vi "dfd_SOS Gain Distribution.vi"(7 "power of 2 initial?":bool, 9 "coefficients b":dbl[](array[numeric]), 10 "initial":dbl, 11 "norms":dbl[](array[numeric])) -> (0 "global gain":dbl, 1 "scaled coefficients b":dbl[](array[numeric]), 3 "input shift":i16)   [LabVIEW 2017, in "NI_DigFilter_FXP.lvlib"]
uses:
  <vilib>/addons/Digital Filter Design/NI_DigFilter_FXP.lvlib
  <vilib>/addons/Digital Filter Design/NI_DigFilterLicensed.lvlib
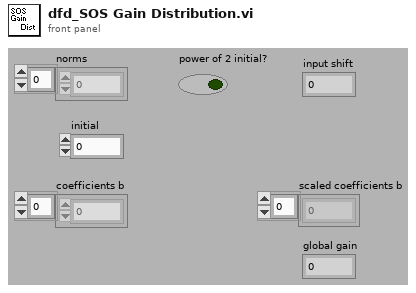
[diagram p1: front panel]
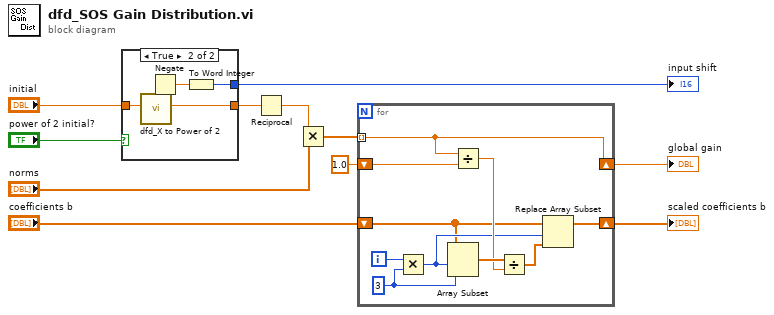
[diagram p0: block diagram]
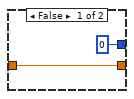
[diagram p2: hidden frame]
diagram:
  n1 = case shown="True" "power of 2 initial?" {
    tunnel: "initial" -> [w12 w18]
    tunnel: [i16 0 w15] -> w6
    tunnel: [w12 w14] -> w5
    frame False {
    }
    frame True {
      n2 = call <vilib>:"dfd_X to Power of 2.vi"("x"=w18) -> ("2^n x"=w14:dbl, "n"=w17:dbl)  [unwired: 9 out]
      n3 = Negate(x=w17) -> (-x=w16:dbl)
      n4 = To Word Integer(number=w16) -> (16bit integer=w15:i16)
    }
  }
  "input shift" <- w6
  n5 = Reciprocal(x=w5) -> (1/x=w3:dbl)
  n6 = Multiply(x=w3, y="norms") -> (x*y=w4:dbl[])
  n7 = for {
    tunnel: w4 -> [w25] mode=indexing
    shift-right: [w25] -> w11
    shift-left: 1.0 -> [w24]
    shift-right: [w22] -> w10
    shift-left: "coefficients b" -> [w19]
    i -> [w27]
    w28 = 3
    n8 = Multiply(x=w27, y=w28) -> (x*y=w21:i32)
    n9 = Array Subset(array=w19, index=w21, length=w28) -> (w26:dbl[])
    n10 = Divide(x=w25, y=w24) -> (x/y=w23:dbl)
    n11 = Divide(x=w26, y=w23) -> (x/y=w20:dbl[])
    n12 = Replace Array Subset(array=w19, new element=w20, index=w21) -> (w22:dbl[])
  }
  "global gain" <- w11
  "scaled coefficients b" <- w10
